vi "RS-422 Transceiver Control.vi"(8 "error in (no error)":errorcluster, 9 "Serial Settings":T1={"baud rate"=9600, "data bits"=8, "parity"=enum."None", "stop bits"=10, "flow control"=0} {"flow control" items=["None"=0, "XON/XOFF"=1, "RTS/CTS"=2, "DTR/DSR"=4]; "stop bits" items=["1.0"=10, "1.5"=15, "2.0"=20]; "data bits" min=5 max=8 step=1; "baud rate" items=["75"=75, "110"=110, "134"=134, "150"=150, "300"=300, "600"=600, "1200"=1200, "1800"=1800, "2400"=2400, "4800"=4800, "7200"=7200, "9600"=9600, "14400"=14400, "19200"=19200, "28800"=28800, "38400"=38400, "56000"=56000, "57600"=57600, "115200"=115200, "128000"=128000, "230400"=230400]}, 10 "Write String":string="*IDN?", 11 "VISA RS 485 Resource":refnum<visa-resource-name>="COM1") -> (0 "error out":errorcluster, 2 "Response":string)   [LabVIEW 2017]
doc: "This example sets the RS-485 transceiver control modes for the specified port and performs a serial port read, a serial port write, or a combination of these actions. If all are selected, the VI will write the data first, read data and then close the VISA session that is opened to the port. This VI will wait until the specified number of bytes is received at the port or until a termination character is received. This example will work only with National Instruments RS-485 interfaces.\n\nThis example demonstrates the transceiver control modes available when using a National Instruments RS-485 product. When connecting one or several devices via RS-485, a user may want to cut down on the amount of wiring. Alternatively, some devices offer a certain wiring configuration that you may need to match. Determine the wiring needs of the connected serial device to determine which NI RS-485 transceiver control mode to choose.\n\nWhen you are communicating with a two-wire device, National Instruments recommends that you use the two-wire Auto Control mode. This mode handles the transmitter/receiver enabling for a two-wire connection in your hardware, so it reduces the software overhead required to perform this operation in your application program."
uses:
  Serial - Settings.ctl
  <vilib>/Instr/_visa.llb/VISA Configure Serial Port (Instr).vi
panel:
  in  "Termination Character":u8=10 format="%.0x"
  in  "End Write on Termination Character?":bool=TRUE
  in  "End Read on Termination Character?":bool=TRUE
  in  "RS-485 Transceiver Mode":u16(ring) items=["Wire4", "Wire2-EchoDTR", "Wire2-CtrlDTR", "Wire2-Auto"]
  in  "Assert DTR?":bool
  # "Overview: Demonstrates the use of the VISA functions to configure NI RS-485 hardware.\nRequirements: NI-Serial and NI-VISA Drivers, NI RS-485 hardware\nInstructions:\n1. Ensure the resource specified in the VISA RS 485 Resource control is a valid NI RS-485 device, and that the Assert DTR? value is correct for your device.\n2. Specify the proper RS-485 Transceiver Mode value for your device.\n3. Run the VI.\n4. View the Response returned by the device."
  # "0xA is equivalent to a '\\n' character, which is a line feed."
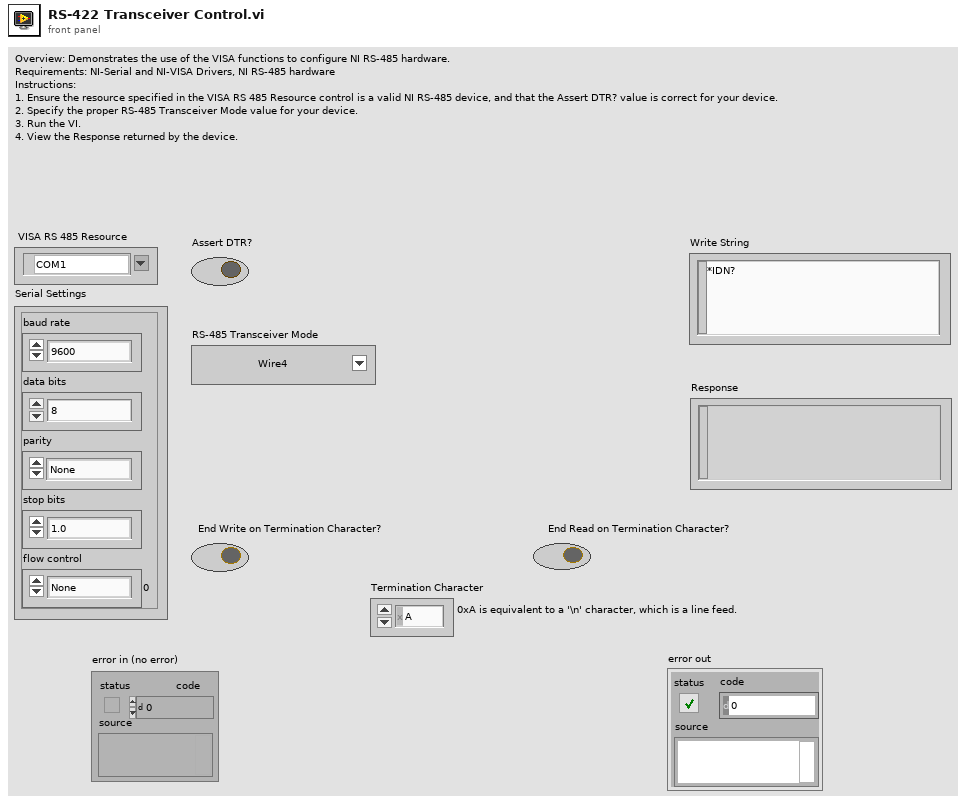
[diagram p1: front panel]
types:
  T1 = typedef "Serial - Settings.ctl" = cluster{"baud rate":u32, "data bits":u16, "parity":enum16{"None", "Odd", "Even", "Mark", "Space"}, "stop bits":u16, "flow control":u16}
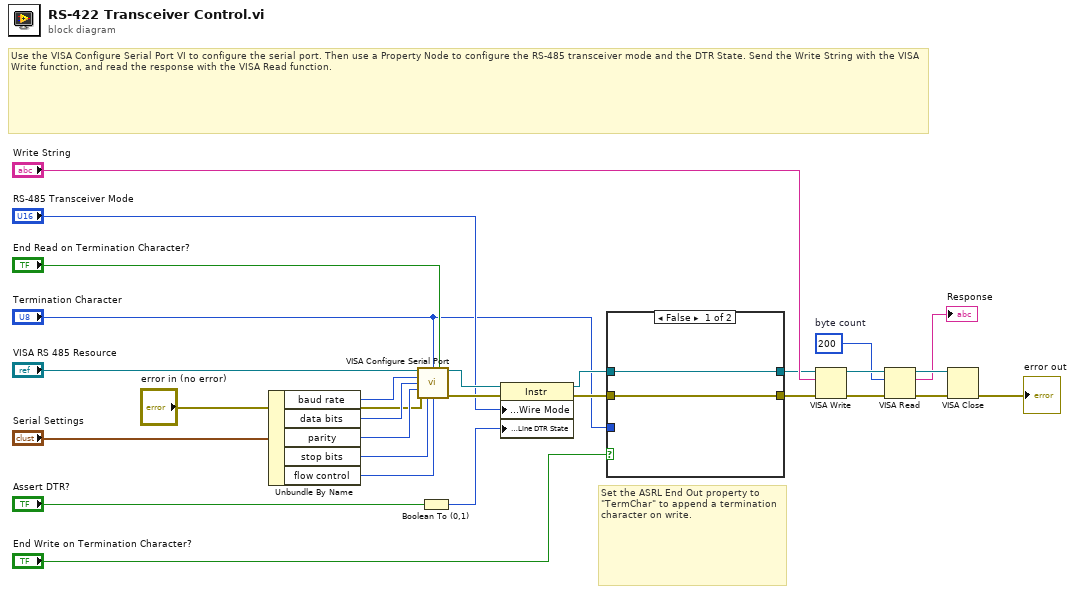
[diagram p0: block diagram]
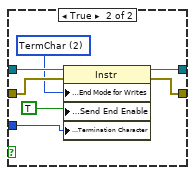
[diagram p2: hidden frame]
diagram:
  w19 = u32 200  # byte count
  # "Set the ASRL End Out property to \"TermChar\" to append a termination character on write."
  # "Use the VISA Configure Serial Port VI to configure the serial port. Then use a Property Node to configure the RS-485 transceiver mode and the DTR State. Send the Write String with the VISA Write function, and read the response with the VISA Read function."
  n1 = Unbundle By Name("Serial Settings") -> ("baud rate"=w16:u32, "data bits"=w15:u16, "parity"=w14:enum16{"None", "Odd", "Even", "Mark", "Space"}, "stop bits"=w13:u16, "flow control"=w12:u16)
  n2 = call-poly "VISA Configure Serial Port"("VISA resource name"="VISA RS 485 Resource", "termination char\n(0xA = '\\n' = LF)"="Termination Character", "Enable Termination\nChar (T)"="End Read on Termination Character?", "baud rate (9600)"=w16, "data bits (8)"=w15, "parity (0:none)"=w14, "error in (no error)"="error in (no error)", "stop bits (10: 1 bit)"=w13, "flow control (0:none)"=w12) -> ("VISA resource name out"=w24:refnum<visa-resource-name>, "error out"=w23:errorcluster)  [unwired: 1 in, 4 out]
  n3 = Boolean To (0,1)(Boolean="Assert DTR?") -> (0, 1=w21:i16)
  n4 = property class="Instr"(reference=w24, error in=w23, "Serial Settings:Wire Mode"="RS-485 Transceiver Mode", "Serial Settings:Modem Line Settings:Line DTR State"=w21) -> (reference out=w6:refnum<visa-resource-name>, error out=w7:errorcluster)
  n5 = case shown="False" "End Write on Termination Character?" {
    tunnel: w6 -> [w29 w37]
    tunnel: w7 -> [w30 w36]
    tunnel: [w29 w35] -> w5
    tunnel: [w30 w34] -> w8
    tunnel: "Termination Character" -> [_ w32]
    frame False {
    }
    frame True {
      w33 = u16 2 items=["None", "LastBit", "TermChar", "Break"] ("Serial Settings:Serial End Mode for Writes")
      n6 = property class="Instr"(reference=w37, error in=w36, "Serial Settings:End Mode for Writes"=w33, "Message Based Settings:Send End Enable"=TRUE, "Message Based Settings:Termination Character"=w32) -> (reference out=w35:refnum<visa-resource-name>, error out=w34:errorcluster)
    }
  }
  n7 = VISA Write(VISA resource name=w5, write buffer="Write String", error in (no error)=w8) -> (VISA resource name out=w27:refnum<visa-resource-name>, error out=w20:errorcluster)  [unwired: 1 out]
  n8 = VISA Read(VISA resource name=w27, byte count=w19, error in (no error)=w20) -> (VISA resource name out=w25:refnum<visa-resource-name>, read buffer=→"Response":string, error out=w26:errorcluster)  [unwired: 1 out]
  n9 = VISA Close(VISA resource name=w25, error in (no error)=w26) -> (error out=→"error out":errorcluster)
